vi "Global 1.vi"() -> ()   [LabVIEW 2019]
panel:
  in  "Array":dbl[](array[numeric])
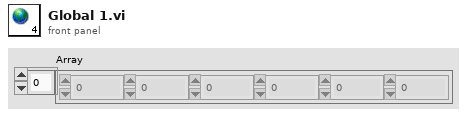
[diagram p1: front panel]
diagram:
